vi "Update zone indicators.vi"(8 "error in (no error)":errorcluster, 10 "Zone Indicators.Timing":sgl, 11 "Application Data in":T1 {"Water Pressure Sensor (%)" scale=0.0..100.0}) -> (0 "error out":errorcluster, 3 "Application Data out":T1 {"Water Pressure Sensor (%)" scale=0.0..100.0})   [LabVIEW 2019]
uses:
  Controls/Application Data.ctl
  Controls/Zone Indicators.ctl
  Controls/Controller Status.ctl
  Controls/Zone Setup Array.ctl
  Controls/Water Pressure Sensor.ctl
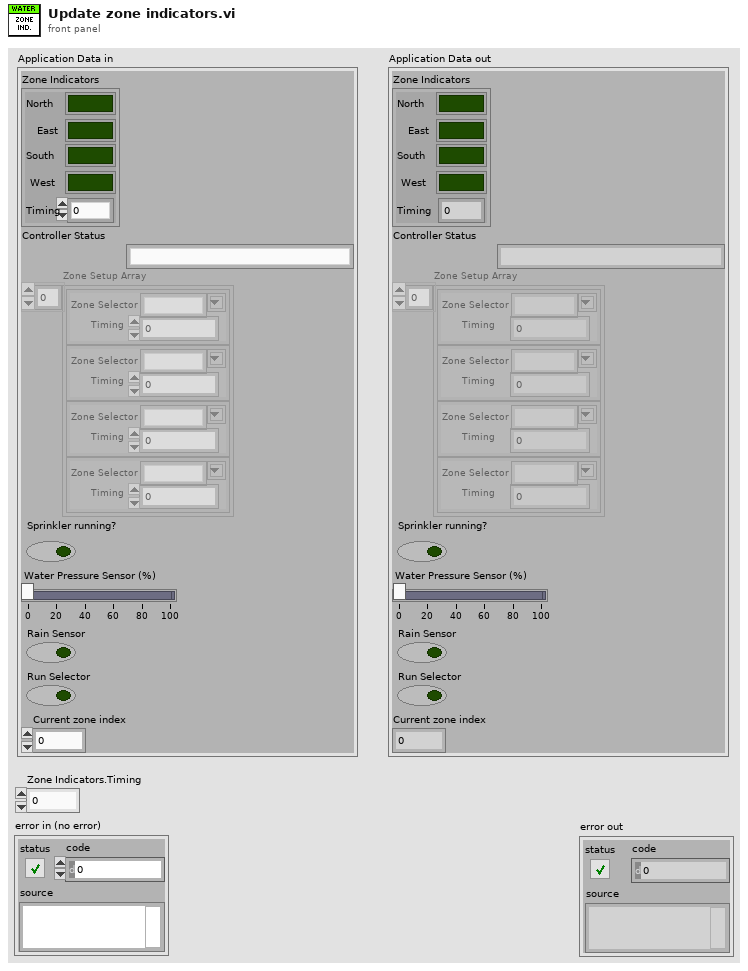
[diagram p1: front panel]
types:
  T1 = typedef "Application Data.ctl" = cluster{"Zone Indicators":T2, "Controller Status":T3, "Zone Setup Array":T4, "Sprinkler running?":bool, "Water Pressure Sensor (%)":T5, "Rain Sensor":bool, "Run Selector":bool, "Current zone index":i32}
  T2 = typedef "Zone Indicators.ctl" = cluster{"North":bool, "East":bool, "South":bool, "West":bool, "Timing":sgl}
  T3 = typedef "Controller Status.ctl" = string
  T4 = typedef "Zone Setup Array.ctl" = cluster{"Zone Selector":string, "Timing":dbl}[]
  T5 = typedef "Water Pressure Sensor.ctl" = u32
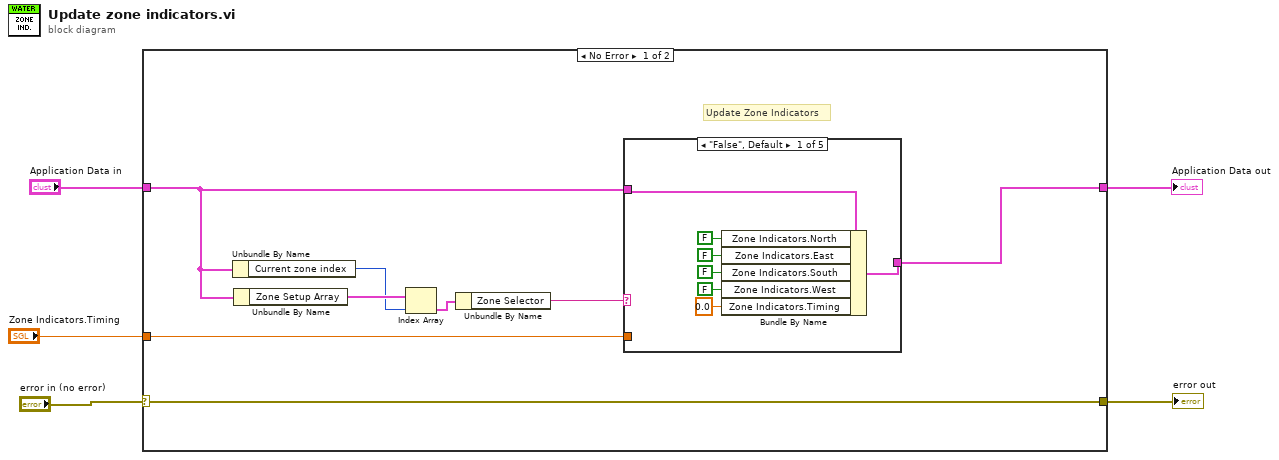
[diagram p0: block diagram]
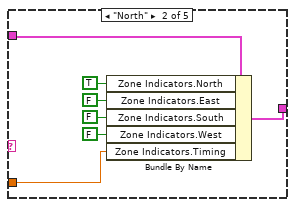
[diagram p2: hidden frame]
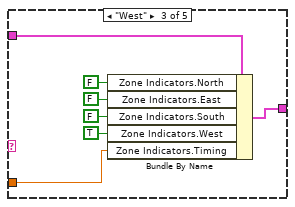
[diagram p3: hidden frame]
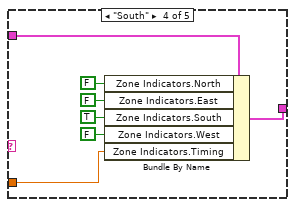
[diagram p4: hidden frame]
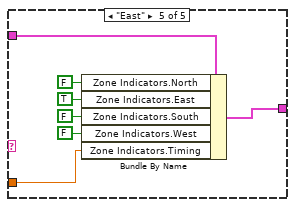
[diagram p5: hidden frame]
diagram:
  n1 = case shown="No Error" "error in (no error)" {
    selector: "error in (no error)" -> [w9 w50]
    tunnel: [w9 w50] -> w4
    tunnel: "Application Data in" -> [w8 w49]
    tunnel: [w7 w49] -> w2
    tunnel: "Zone Indicators.Timing" -> [w6 _]
    frame No Error {
      # "Update Zone Indicators"
      n2 = Unbundle By Name(w8) -> ("Current zone index"=w10:i32)
      n3 = Unbundle By Name(w8) -> ("Zone Setup Array"=w11:T4)
      n4 = Index Array(array=w11, index=w10) -> (element=w12:cluster{"Zone Selector":string, "Timing":dbl})
      n5 = Unbundle By Name(w12) -> ("Zone Selector"=w13:string)
      n6 = case shown="\"False\", Default" w13 {
        tunnel: w8 -> [w16 w23 w30 w37 w48]
        tunnel: [w15 w22 w29 w36 w43] -> w7
        tunnel: w6 -> [_ w21 w28 w35 w42]
        frame "False", Default {
          n7 = Bundle By Name(cluster=w16, "Zone Indicators.North"=FALSE, "Zone Indicators.East"=FALSE, "Zone Indicators.South"=FALSE, "Zone Indicators.West"=FALSE, "Zone Indicators.Timing"=sgl 0.0) -> (w15:T1)
        }
        frame "North" {
          n8 = Bundle By Name(cluster=w23, "Zone Indicators.North"=TRUE, "Zone Indicators.East"=FALSE, "Zone Indicators.South"=FALSE, "Zone Indicators.West"=FALSE, "Zone Indicators.Timing"=w21) -> (w22:T1)
        }
        frame "West" {
          n9 = Bundle By Name(cluster=w30, "Zone Indicators.North"=FALSE, "Zone Indicators.East"=FALSE, "Zone Indicators.South"=FALSE, "Zone Indicators.West"=TRUE, "Zone Indicators.Timing"=w28) -> (w29:T1)
        }
        frame "South" {
          n10 = Bundle By Name(cluster=w37, "Zone Indicators.North"=FALSE, "Zone Indicators.East"=FALSE, "Zone Indicators.South"=TRUE, "Zone Indicators.West"=FALSE, "Zone Indicators.Timing"=w35) -> (w36:T1)
        }
        frame "East" {
          n11 = Bundle By Name(cluster=w48, "Zone Indicators.North"=FALSE, "Zone Indicators.East"=TRUE, "Zone Indicators.South"=FALSE, "Zone Indicators.West"=FALSE, "Zone Indicators.Timing"=w42) -> (w43:T1)
        }
      }
    }
    frame Error {
    }
  }
  "error out" <- w4
  "Application Data out" <- w2
